vi "Discrete Limited Integrator (DBL Array).vi"(0 "input points":dbl[](array[numeric]) format="%.2f", 1 "initial conditions":dbl[](array[numeric]) format="%.2f", 3 "bounds":cluster{"upper bound":dbl, "lower bound":dbl}[](array[cluster]) {"lower bound" format="%.2f"; "upper bound" format="%.2f"}, 4 "initialize":bool) -> (5 "output points":dbl[](array[numeric]) format="%.2f")   [LabVIEW 2020, in "NI_AdvCtrl_discrete linear.lvlib"]
doc: "LabVIEW no longer supports this VI. You can obtain similar functionality by installing the LabVIEW Simulation Module.\n\nIntegrates a discrete input signal. The result of the discrete integration is limited by the lower and upper bound."
uses:
  <vilib>/addons/control/advanced/NI_AdvCtrl_discrete linear.lvlib
  <vilib>/addons/control/advanced/NI_AdvCtrl_continuous linear.lvlib
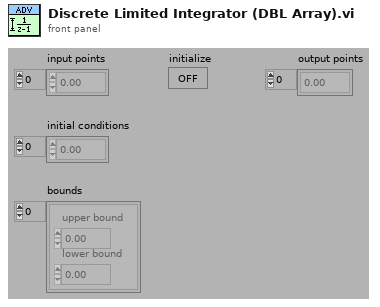
[diagram p1: front panel]
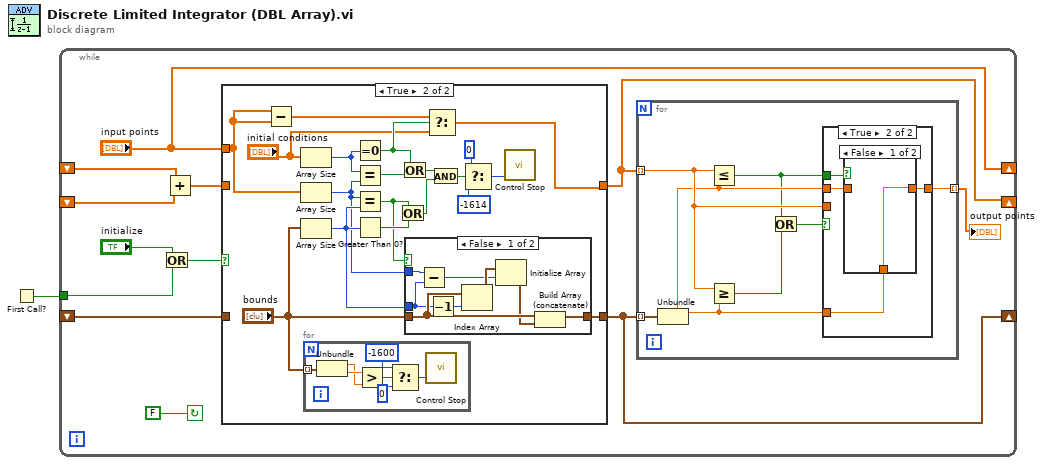
[diagram p0: block diagram]
diagram:
  n1 = First Call?() -> (First Call?: T/F=w1:bool)
  n2 = while {
    shift-left: _ -> [w6]
    shift-right: [w5] -> _
    shift-left: _ -> [w2]
    shift-right: ["input points"] -> _
    tunnel: w1 -> [w11]
    shift-left: _ -> [w9]
    shift-right: [w4] -> _
    stop <- FALSE continue-if-true
    n3 = Or(x="initialize", y=w11) -> (x .or. y?=w10:bool)
    n4 = Add(x=w2, y=w9) -> (x+y=w8:dbl[])
    n5 = case shown="True" w10 {
      tunnel: "input points" -> [_ w41]
      tunnel: [w29 w42] -> w4
      tunnel: w8 -> [w29 _]
      tunnel: [w30 w34] -> w5
      tunnel: w6 -> [w30 _]
      frame False {
      }
      frame True {
        n6 = Subtract(x=w41, y=w41) -> (x-y=w40:dbl[])
        n7 = Array Size(array="initial conditions") -> (size(s)=w45:i32)
        n8 = Array Size(array=w41) -> (size(s)=w32:i32)
        n9 = Array Size(array="bounds") -> (size(s)=w33:i32)
        n10 = for {
          tunnel: "bounds" -> [w56] mode=indexing
          n11 = Unbundle(w56) -> ("upper bound"=w51:dbl, "lower bound"=w52:dbl)
          n12 = Greater?(x=w52, y=w51) -> (0:w55:bool)
          n13 = Select(t=-1600, s=w55, f=0) -> (s? t:f=w53:i32)
          n14 = call <vilib>:"Control Stop.vi"("error"=w53) -> ()  [unwired: 2 out]
        }
        n15 = Equal To 0?(x=w45) -> (x = 0?=w44:bool)
        n16 = Equal?(x=w45, y=w32) -> (x = y?=w46:bool)
        n17 = Equal?(x=w32, y=w33) -> (x = y?=w35:bool)
        n18 = Greater Than 0?(x=w33) -> (x > 0?=w36:bool)
        n19 = Or(x=w35, y=w36) -> (x .or. y?=w37:bool)
        n20 = Or(x=w44, y=w46) -> (x .or. y?=w38:bool)
        n21 = case shown="False" w35 {
          tunnel: [w64 w65] -> w34
          tunnel: "bounds" -> [w63 w65]
          tunnel: w33 -> [w58 _]
          tunnel: w32 -> [w59 _]
          frame False {
            n22 = Subtract(x=w59, y=w58) -> (x-y=w57:i32)
            n23 = Decrement(x=w58) -> (x-1=w62:i32)
            n24 = Index Array(array=w63, index=w62) -> (element=w61:cluster{"upper bound":dbl, "lower bound":dbl})
            n25 = Initialize Array(w61, w57) -> (w60:cluster{"upper bound":dbl, "lower bound":dbl}[])
            n26 = Build Array (concatenate)(w63, w60) -> (w64:cluster{"upper bound":dbl, "lower bound":dbl}[])
          }
          frame True {
          }
        }
        n27 = Select(t=w40, s=w44, f="initial conditions") -> (s? t:f=w42:dbl[])
        n28 = And(x=w38, y=w37) -> (x .and. y?=w39:bool)
        n29 = Select(t=0, s=w39, f=-1614) -> (s? t:f=w49:i32)
        n30 = call <vilib>:"Control Stop.vi"("error"=w49) -> ()  [unwired: 2 out]
      }
    }
    n31 = for {
      tunnel: [w20] -> w3 mode=indexing
      tunnel: w4 -> [w19] mode=indexing
      tunnel: w5 -> [w18] mode=indexing
      n32 = Unbundle(w18) -> ("upper bound"=w17:dbl, "lower bound"=w16:dbl)
      n33 = Less Or Equal?(x=w19, y=w16) -> (x <= y?=w14:bool)
      n34 = Greater Or Equal?(x=w19, y=w17) -> (x >= y?=w15:bool)
      n35 = Or(x=w14, y=w15) -> (x .or. y?=w21:bool)
      n36 = case shown="True" w21 {
        tunnel: [w22 w24] -> w20
        tunnel: w19 -> [w22 _]
        tunnel: w14 -> [_ w26]
        tunnel: w16 -> [_ w25]
        tunnel: w17 -> [_ w23]
        frame False {
        }
        frame True {
          n37 = case shown="False" w26 {
            tunnel: w25 -> [_ w28]
            tunnel: [w27 w28] -> w24
            tunnel: w23 -> [w27 _]
            frame False {
            }
            frame True {
            }
          }
        }
      }
    }
    "output points" <- w3
  }
